vi "Read Stand_relays.vi"(8 "error in (no error)":errorcluster, 11 "Algorythm in":refnum<class "Algorythm.lvclass">) -> (0 "error out":errorcluster, 2 "Stand_relays":refnum<vi>, 3 "Algorythm out":refnum<class "Algorythm.lvclass">)   [LabVIEW 2020, in "Algorythm.lvlib" / "Algorythm.lvclass"]
uses:
  Algorythm.lvclass
  Algorythm.lvclass/Algorythm.ctl
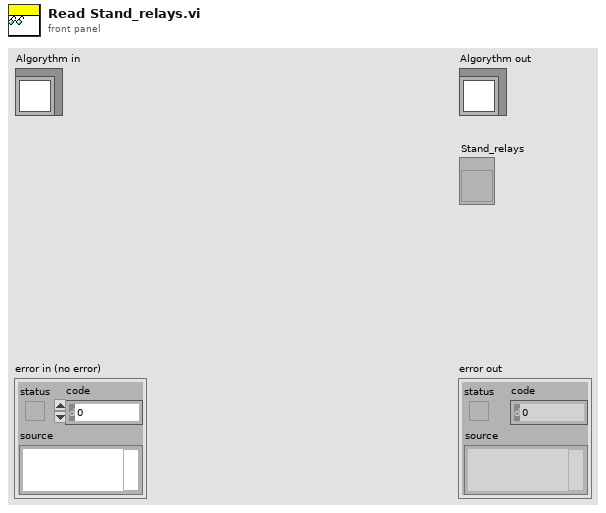
[diagram p1: front panel]
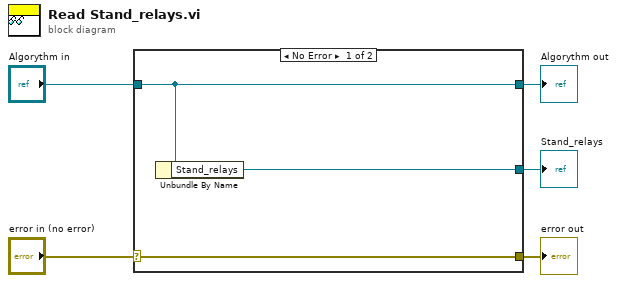
[diagram p0: block diagram]
diagram:
  n1 = case shown="No Error" "error in (no error)" {
    selector: "error in (no error)" -> [w8 w9]
    tunnel: [w8 w9] -> w4
    tunnel: [w7 w10] -> w2
    tunnel: "Algorythm in" -> [w7 w10]
    tunnel: [w6 _] -> w1
    frame No Error {
      n2 = Unbundle By Name(w7) -> ("Stand_relays"=w6:refnum<vi>)
    }
    frame Error {
    }
  }
  "error out" <- w4
  "Algorythm out" <- w2
  "Stand_relays" <- w1
